vi "Update FIFO Address - 32-bit Address.vi"(0 "address in":u32, 5 "increment":bool, 7 "fifo depth":T1=10 items=["4"=2, "8"=3, "16"=4, "32"=5, "64"=6, "128"=7, "256"=8, "512"=9, "1024"=10, "2048"=11, "4096"=12, "8192"=13, "16384"=14, "32768"=15, "65536"=16, "131072"=17, "262144"=18, "524288"=19, "1048576"=20, "2097152"=21, "4194304"=22, "8388608"=23, "16777216"=24, "33554432"=25, "67108864"=26, "134217728"=27, "268435456"=28, "536870912"=29, "1073741824"=30, "2147483648"=31, "4294967296"=32]) -> (4 "address out":u32)   [LabVIEW 2012, in "FIFO.lvlib"]
uses:
  <userlib>/FPGA Library/Code Development/DRAM/RF-RIO/FIFO/FIFO/FPGA/FIFO.lvlib
  <userlib>/FPGA Library/Code Development/DRAM/RF-RIO/FIFO/FIFO/FPGA/Private/FIFO Depth - 32-bit Address.ctl
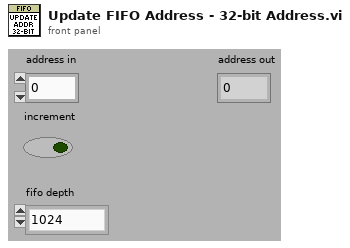
[diagram p1: front panel]
types:
  T1 = typedef "FIFO.lvlib/FIFO Depth - 32-bit Address.ctl" = u8
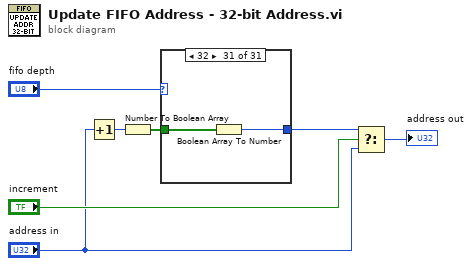
[diagram p0: block diagram]
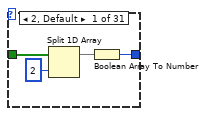
[diagram p2: hidden frame]
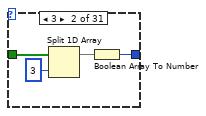
[diagram p3: hidden frame]
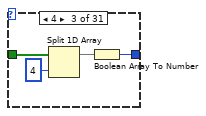
[diagram p4: hidden frame]
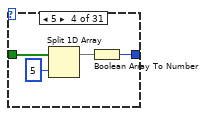
[diagram p5: hidden frame]
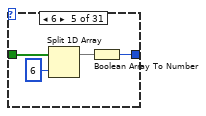
[diagram p6: hidden frame]
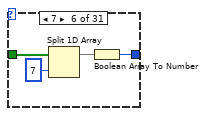
[diagram p7: hidden frame]
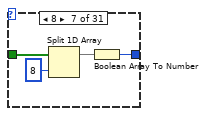
[diagram p8: hidden frame]
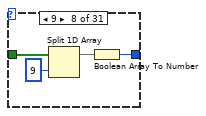
[diagram p9: hidden frame]
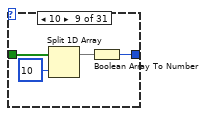
[diagram p10: hidden frame]
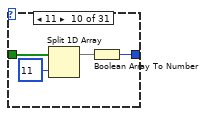
[diagram p11: hidden frame]
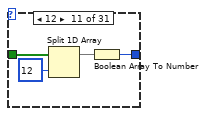
[diagram p12: hidden frame]
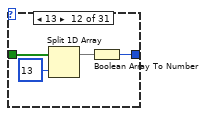
[diagram p13: hidden frame]
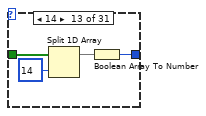
[diagram p14: hidden frame]
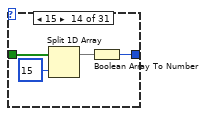
[diagram p15: hidden frame]
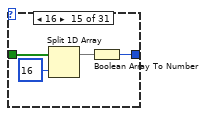
[diagram p16: hidden frame]
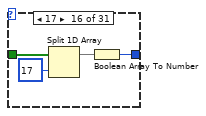
[diagram p17: hidden frame]
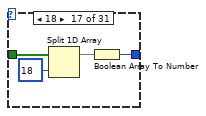
[diagram p18: hidden frame]
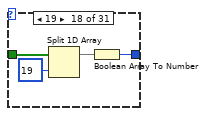
[diagram p19: hidden frame]
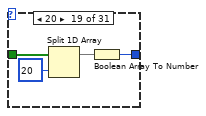
[diagram p20: hidden frame]
diagram:
  n1 = Increment(x="address in") -> (x+1=w2:u32)
  n2 = Number To Boolean Array(number=w2) -> (Boolean array=w1:bool[])
  n3 = case shown="32" "fifo depth" {
    tunnel: w1 -> [w10 w14 w18 w22 w26 w30 w34 w38 w42 w46 w50 w54 w58 w62 w66 w70 w74 w78 w82 w86 w90 w94 w98 w102 w106 w110 w114 w118 w122 w126 w128]
    tunnel: [w11 w15 w19 w23 w27 w31 w35 w39 w43 w47 w51 w55 w59 w63 w67 w71 w75 w79 w83 w87 w91 w95 w99 w103 w107 w111 w115 w119 w123 w127 w129] -> w5
    frame 2, Default {
      n4 = Split 1D Array(array=w10, index=2) -> (first subarray=w8:bool[])  [unwired: 1 out]
      n5 = Boolean Array To Number(Boolean array=w8) -> (number=w11:u32)
    }
    frame 3 {
      n6 = Split 1D Array(array=w14, index=3) -> (first subarray=w12:bool[])  [unwired: 1 out]
      n7 = Boolean Array To Number(Boolean array=w12) -> (number=w15:u32)
    }
    frame 4 {
      n8 = Split 1D Array(array=w18, index=4) -> (first subarray=w16:bool[])  [unwired: 1 out]
      n9 = Boolean Array To Number(Boolean array=w16) -> (number=w19:u32)
    }
    frame 5 {
      n10 = Split 1D Array(array=w22, index=5) -> (first subarray=w20:bool[])  [unwired: 1 out]
      n11 = Boolean Array To Number(Boolean array=w20) -> (number=w23:u32)
    }
    frame 6 {
      n12 = Split 1D Array(array=w26, index=6) -> (first subarray=w24:bool[])  [unwired: 1 out]
      n13 = Boolean Array To Number(Boolean array=w24) -> (number=w27:u32)
    }
    frame 7 {
      n14 = Split 1D Array(array=w30, index=7) -> (first subarray=w28:bool[])  [unwired: 1 out]
      n15 = Boolean Array To Number(Boolean array=w28) -> (number=w31:u32)
    }
    frame 8 {
      n16 = Split 1D Array(array=w34, index=8) -> (first subarray=w32:bool[])  [unwired: 1 out]
      n17 = Boolean Array To Number(Boolean array=w32) -> (number=w35:u32)
    }
    frame 9 {
      n18 = Split 1D Array(array=w38, index=9) -> (first subarray=w36:bool[])  [unwired: 1 out]
      n19 = Boolean Array To Number(Boolean array=w36) -> (number=w39:u32)
    }
    frame 10 {
      n20 = Split 1D Array(array=w42, index=10) -> (first subarray=w40:bool[])  [unwired: 1 out]
      n21 = Boolean Array To Number(Boolean array=w40) -> (number=w43:u32)
    }
    frame 11 {
      n22 = Split 1D Array(array=w46, index=11) -> (first subarray=w44:bool[])  [unwired: 1 out]
      n23 = Boolean Array To Number(Boolean array=w44) -> (number=w47:u32)
    }
    frame 12 {
      n24 = Split 1D Array(array=w50, index=12) -> (first subarray=w48:bool[])  [unwired: 1 out]
      n25 = Boolean Array To Number(Boolean array=w48) -> (number=w51:u32)
    }
    frame 13 {
      n26 = Split 1D Array(array=w54, index=13) -> (first subarray=w52:bool[])  [unwired: 1 out]
      n27 = Boolean Array To Number(Boolean array=w52) -> (number=w55:u32)
    }
    frame 14 {
      n28 = Split 1D Array(array=w58, index=14) -> (first subarray=w56:bool[])  [unwired: 1 out]
      n29 = Boolean Array To Number(Boolean array=w56) -> (number=w59:u32)
    }
    frame 15 {
      n30 = Split 1D Array(array=w62, index=15) -> (first subarray=w60:bool[])  [unwired: 1 out]
      n31 = Boolean Array To Number(Boolean array=w60) -> (number=w63:u32)
    }
    frame 16 {
      n32 = Split 1D Array(array=w66, index=16) -> (first subarray=w64:bool[])  [unwired: 1 out]
      n33 = Boolean Array To Number(Boolean array=w64) -> (number=w67:u32)
    }
    frame 17 {
      n34 = Split 1D Array(array=w70, index=17) -> (first subarray=w68:bool[])  [unwired: 1 out]
      n35 = Boolean Array To Number(Boolean array=w68) -> (number=w71:u32)
    }
    frame 18 {
      n36 = Split 1D Array(array=w74, index=18) -> (first subarray=w72:bool[])  [unwired: 1 out]
      n37 = Boolean Array To Number(Boolean array=w72) -> (number=w75:u32)
    }
    frame 19 {
      n38 = Split 1D Array(array=w78, index=19) -> (first subarray=w76:bool[])  [unwired: 1 out]
      n39 = Boolean Array To Number(Boolean array=w76) -> (number=w79:u32)
    }
    frame 20 {
      n40 = Split 1D Array(array=w82, index=20) -> (first subarray=w80:bool[])  [unwired: 1 out]
      n41 = Boolean Array To Number(Boolean array=w80) -> (number=w83:u32)
    }
    frame 21 {
      n42 = Split 1D Array(array=w86, index=21) -> (first subarray=w84:bool[])  [unwired: 1 out]
      n43 = Boolean Array To Number(Boolean array=w84) -> (number=w87:u32)
    }
    frame 22 {
      n44 = Split 1D Array(array=w90, index=22) -> (first subarray=w88:bool[])  [unwired: 1 out]
      n45 = Boolean Array To Number(Boolean array=w88) -> (number=w91:u32)
    }
    frame 23 {
      n46 = Split 1D Array(array=w94, index=23) -> (first subarray=w92:bool[])  [unwired: 1 out]
      n47 = Boolean Array To Number(Boolean array=w92) -> (number=w95:u32)
    }
    frame 24 {
      n48 = Split 1D Array(array=w98, index=24) -> (first subarray=w96:bool[])  [unwired: 1 out]
      n49 = Boolean Array To Number(Boolean array=w96) -> (number=w99:u32)
    }
    frame 25 {
      n50 = Split 1D Array(array=w102, index=25) -> (first subarray=w100:bool[])  [unwired: 1 out]
      n51 = Boolean Array To Number(Boolean array=w100) -> (number=w103:u32)
    }
    frame 26 {
      n52 = Split 1D Array(array=w106, index=26) -> (first subarray=w104:bool[])  [unwired: 1 out]
      n53 = Boolean Array To Number(Boolean array=w104) -> (number=w107:u32)
    }
    frame 27 {
      n54 = Split 1D Array(array=w110, index=27) -> (first subarray=w108:bool[])  [unwired: 1 out]
      n55 = Boolean Array To Number(Boolean array=w108) -> (number=w111:u32)
    }
    frame 28 {
      n56 = Split 1D Array(array=w114, index=28) -> (first subarray=w112:bool[])  [unwired: 1 out]
      n57 = Boolean Array To Number(Boolean array=w112) -> (number=w115:u32)
    }
    frame 29 {
      n58 = Split 1D Array(array=w118, index=29) -> (first subarray=w116:bool[])  [unwired: 1 out]
      n59 = Boolean Array To Number(Boolean array=w116) -> (number=w119:u32)
    }
    frame 30 {
      n60 = Split 1D Array(array=w122, index=30) -> (first subarray=w120:bool[])  [unwired: 1 out]
      n61 = Boolean Array To Number(Boolean array=w120) -> (number=w123:u32)
    }
    frame 31 {
      n62 = Split 1D Array(array=w126, index=31) -> (first subarray=w124:bool[])  [unwired: 1 out]
      n63 = Boolean Array To Number(Boolean array=w124) -> (number=w127:u32)
    }
    frame 32 {
      n64 = Boolean Array To Number(Boolean array=w128) -> (number=w129:u32)
    }
  }
  n65 = Select(t=w5, s="increment", f="address in") -> (s? t:f=→"address out":u32)
